vi "Horsterei.vi"() -> ()   [LabVIEW 2017]
uses:
  <vilib>/rvi/interface/nirviMethod/nirviMethod.xnode
  E:/HAGAR-V_ECD/FPGA-Programm_ECD.vi
  <vilib>/FPGAPlugInAG/cRIO-9035/niLvFpga_WriteFifo_cRIO-9035.vi
  <vilib>/rvi/errors/niLvFpgaMergeErrorWithErrorCode.vi
  <vilib>/FPGAPlugInAG/cRIO-9035/niLvFpga_ReadFifo_cRIO-9035.vi
  <vilib>/rvi/interface/nirviReadWriteControl/nirviReadWriteControl.xnode
  <vilib>/rvi/interface/nirviCloseFPGA/nirviCloseFPGA.xnode
  FPGA Bitfiles/HAGAR-VECD_FPGATarget_FPGA-ProgrammECD_J-wKM9Jb3G8.lvbitx
  NiFpgaLv.dll
  <vilib>/Utility/error.llb/Error Cluster From Error Code.vi
  <vilib>/rvi/errors/niLvFpgaAdjustHostInterfaceError.vi
  <vilib>/FPGAPlugInAG/cRIO-9035/niLvFpga_Close_cRIO-9035.vi
panel:
  in  "Numerisch":i32
  in  "SPsenden":bool=TRUE
  in  "SP":u32[](array[numeric])
  in  "SPvorgeben":string[](array[string])=[":0622010121\n", ":0621010121", ":0626010121", ":0620010121", ":0624010121", ":0625010121", ":0623010121"]
  in  "SPquittieren":string[](array[string])=[":0422000005\n", ":0421000005", ":0426000005", ":0420000005", ":0424000005", ":0425000005", ":0423000005"]
  out "MW":u32[](array[numeric])
  in  "MWmitteilen":string[](array[string])=[":0622020121", ":0621020121", ":0626020121", ":0620020121", ":0624020121", ":0625020121", ":0623020121"]
  in  "MWabfragen":string[](array[string])=[":06220401210120", ":06210401210120", ":06260401210120", ":06200401210120", ":06240401210120", ":06250401210120", ":06230401210120"]
  out "stop":errorcluster caption="Fehler (Ausgang)"
  out "Fehler (Ausgang)":errorcluster
  in  "Stopp":bool
  out "FPGA-Start":errorcluster caption="error out"
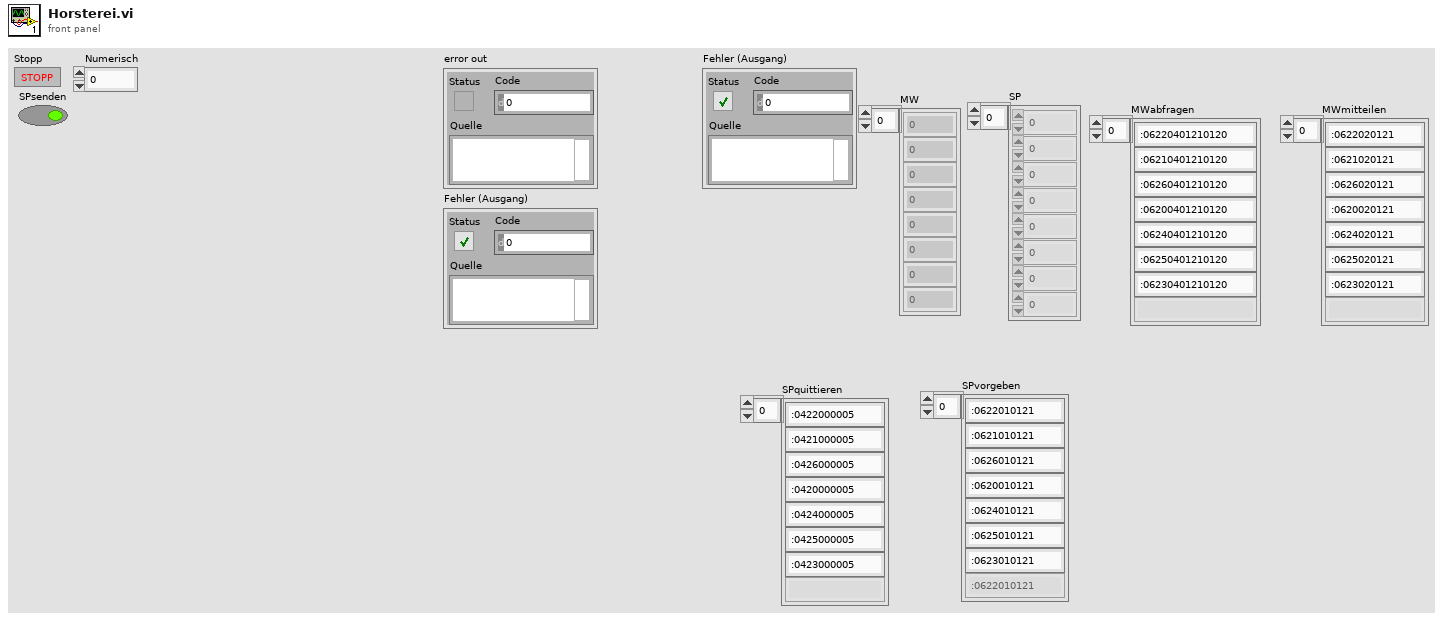
[diagram p1: front panel]
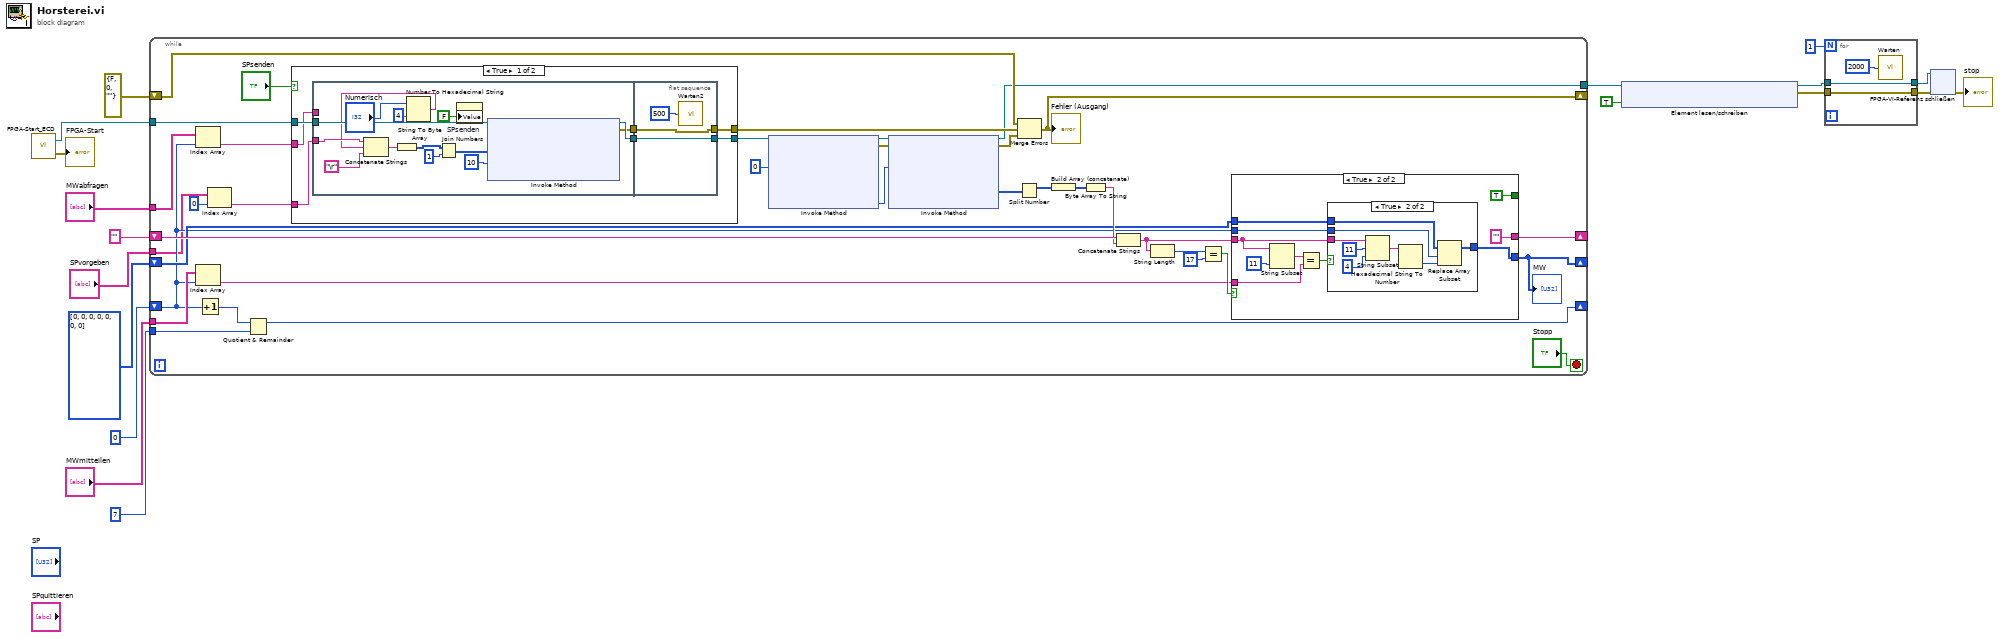
[diagram p0: block diagram]
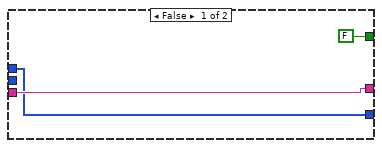
[diagram p2: hidden frame]
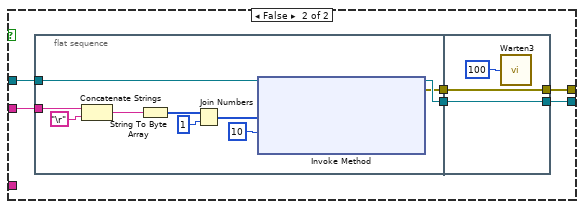
[diagram p4: hidden frame]
diagram:
  n1 = call "FPGA-Start_ECD.vi"() -> ("error out"=→"FPGA-Start":errorcluster, "FPGA-VI-Referenz (Ausgang)"=w18:refnum<k20>)  [unwired: 2 in]
  n2 = while {
    tunnel: w18 -> [w27]
    shift-right: [w46] -> _
    shift-left: errorcluster {"status"=FALSE, "code"=0, "source"=""} ("error IO") -> [w54]
    shift-right: [w34] -> _
    shift-left: "" -> [w42]
    tunnel: [w40] -> w14
    tunnel: "MWabfragen" -> [w33]
    tunnel: "MWmitteilen" -> [w32]
    shift-right: [w30] -> _
    shift-left: u32[] [0, 0, 0, 0, 0, 0, 0] ("MW") -> [w31]
    shift-right: [w22] -> _
    shift-left: 0 -> [w24]
    tunnel: 7 ("y") -> [w23]
    tunnel: "SPvorgeben" -> [w21]
    stop <- "Stopp" stop-if-true
    n3 = Index Array(array=w33, index=w24) -> (element=w29:string)
    n4 = Index Array(array=w32, index=w24) -> (element=w35:string)
    n5 = Increment(x=w24) -> (x+1=w25:i32)
    n6 = Index Array(array=w21, index=0 ("Index")) -> (element=w19:string)
    n7 = Quotient & Remainder(x=w25, y=w23) -> (x-y*floor(x/y)=w22:i32)  [unwired: 1 out]
    n8 = case shown="True" "SPsenden" {
      tunnel: w27 -> [w83 w106]
      tunnel: [w82 w105] -> w52
      tunnel: w29 -> [w81 w104]
      tunnel: [w80 w103] -> w53
      tunnel: w19 -> [w77 _]
      frame True {
        n9 = flat-sequence {
          tunnel: w83 -> [w91]
          tunnel: w81 -> [_]
          tunnel: [w90] -> w79
          tunnel: [w89] -> w78
          tunnel: w77 -> [w88]
          tunnel: [w99] -> w80
          tunnel: [w100] -> w82
          tunnel: w79 -> [w100]
          tunnel: w78 -> [w99]
          frame #0 {
            n10 = Number To Hexadecimal String(1:i16 4 ("Breite (-)"), 2:"Numerisch") -> (0:w85:string)
            n11 = Concatenate Strings(w88, w85, "\r") -> (w92:string)
            n12 = String To Byte Array(string=w92) -> (unsigned byte array=w97:u8[])
            n13 = Join Numbers(hi=w97, lo=u8 1) -> ((hi.lo)=w95:u16[])
            n14 = property on="SPsenden" class="Bool. (strikt)"("Value"=FALSE ("SPsenden")) -> ()  [unwired: 2 in, 2 out]
            n15 = xnode "Invoke Method"("FPGA-VI-Referenz (Eingang)"=w91, "Daten"=w95, "Timeout (ms)"=10) -> ("FPGA-VI-Referenz (Ausgang)"=w90:refnum<k20>, "Fehler (Ausgang)"=w89:errorcluster)  [unwired: 1 in, 1 out]
          }
          frame #1 {
            n16 = call "Warten2"("Count(mSec)"=u32 500) -> ()  [unwired: 1 out]
          }
        }
      }
      frame False {
        n17 = flat-sequence {
          tunnel: w106 -> [w110]
          tunnel: w104 -> [w108]
          tunnel: [w109] -> w102
          tunnel: [w107] -> w101
          tunnel: [w118] -> w103
          tunnel: [w119] -> w105
          tunnel: w102 -> [w119]
          tunnel: w101 -> [w118]
          frame #0 {
            n18 = Concatenate Strings(w108, "\r") -> (w111:string)
            n19 = String To Byte Array(string=w111) -> (unsigned byte array=w116:u8[])
            n20 = Join Numbers(hi=w116, lo=u8 1) -> ((hi.lo)=w114:u16[])
            n21 = xnode "Invoke Method"("FPGA-VI-Referenz (Eingang)"=w110, "Daten"=w114, "Timeout (ms)"=10) -> ("FPGA-VI-Referenz (Ausgang)"=w109:refnum<k20>, "Fehler (Ausgang)"=w107:errorcluster)  [unwired: 1 in, 1 out]
          }
          frame #1 {
            n22 = call "Warten3"("Count(mSec)"=u32 100) -> ()  [unwired: 1 out]
          }
        }
      }
    }
    n23 = xnode "Invoke Method"("FPGA-VI-Referenz (Eingang)"=w52, "Anzahl der Elemente"=u32 0) -> ("FPGA-VI-Referenz (Ausgang)"=w51:refnum<k20>, "Fehler (Ausgang)"=w48:errorcluster, "Verbleibende Elemente"=w49:u32)  [unwired: 2 in, 1 out]
    n24 = xnode "Invoke Method"("FPGA-VI-Referenz (Eingang)"=w51, "Fehler (Eingang)"=w48, "Anzahl der Elemente"=w49) -> ("FPGA-VI-Referenz (Ausgang)"=w40:refnum<k20>, "Fehler (Ausgang)"=w47:errorcluster, "Daten"=w45:u16[])  [unwired: 1 in, 1 out]
    n25 = Merge Errors(w54, w53, w47) -> (w46:errorcluster)
    "Fehler (Ausgang)" <- w46
    n26 = Split Number(x=w45) -> (hi(x)=w44:u8[])  [unwired: 1 out]
    n27 = Build Array (concatenate)(w44) -> (w43:u8[])
    n28 = Byte Array To String(unsigned byte array=w43) -> (string=w39:string)
    n29 = Concatenate Strings(w42, w39) -> (w36:string)
    n30 = String Length(string=w36) -> (length=w38:i32)
    n31 = Equal?(x=w38, y=17) -> (x = y?=w37:bool)
    n32 = case shown="True" w37 {
      tunnel: w36 -> [w57 w65]
      tunnel: w35 -> [_ w59]
      tunnel: [w57 ""] -> w34
      tunnel: [FALSE TRUE] -> _
      tunnel: w31 -> [w55 w62]
      tunnel: w24 -> [_ w58]
      tunnel: [w55 w61] -> w30
      frame False {
      }
      frame True {
        n33 = String Subset(string=w65, length (rest)=11 ("Länge (Rest)")) -> (substring=w67:string)  [unwired: 1 in]
        n34 = Equal?(x=w67, y=w59) -> (x = y?=w66:bool)
        n35 = case shown="True" w66 {
          tunnel: w65 -> [_ w76]
          tunnel: w62 -> [w68 w70]
          tunnel: w58 -> [_ w71]
          tunnel: [w68 w69] -> w61
          frame False {
          }
          frame True {
            n36 = String Subset(string=w76, offset (0)=11 ("Offset (0)"), length (rest)=4 ("Länge (Rest)")) -> (substring=w73:string)
            n37 = Hexadecimal String To Number(string=w73) -> (number=w72:u32)  [unwired: 2 in, 1 out]
            n38 = Replace Array Subset(array=w70, new element=w72, index=w71) -> (w69:u32[])
          }
        }
      }
    }
    "MW" <- w30
  }
  n39 = xnode "Element lesen/schreiben"("FPGA-VI-Referenz (Eingang)"=w14, "global stop"=TRUE) -> ("FPGA-VI-Referenz (Ausgang)"=w12:refnum<k20>, "Fehler (Ausgang)"=w11:errorcluster)  [unwired: 1 in]
  n40 = for {
    N: 1 -> [_]
    tunnel: w12 -> [w121]
    tunnel: w11 -> [w120]
    tunnel: [w121] -> w10
    tunnel: [w120] -> w9
    n41 = call "Warten"("Count(mSec)"=u32 2000) -> ()  [unwired: 1 out]
  }
  n42 = xnode "FPGA-VI-Referenz schließen"("FPGA-VI-Referenz (Eingang)"=w10, "Fehler (Eingang)"=w9) -> ("Fehler (Ausgang)"=→"stop":errorcluster)
